vi "DAQAI_ws.vi"(2 "rate":dbl=1000.0, 3 "number of samples":i32=1000, 4 "timeout (s)":dbl=10.0 format="%0.2f", 5 "error in":errorcluster) -> (15 "data":dynamicdata(graph), 19 "error out":errorcluster)   [LabVIEW 2018]
doc: "Creates, edits, and runs tasks using NI-DAQmx. Refer to the NI-DAQmx Readme for a complete listing of devices NI-DAQmx supports.\n\nWhen you place this Express VI on the block diagram, the DAQ Assistant launches to create a new task. After you create a task, you can double-click the DAQ Assistant Express VI to edit that task. For continuous measurement or generation, place a while loop around the DAQ Assistant Express VI."
uses:
  AI channel settings.ctl
panel:
  in  "stop":bool
  in  "AI channel setting":T1={"device name"="Dev1", "physical channel"=["ai0", "ai1", "ai2", "ai3", "ai4", "ai5", "ai6", "ai7"], "channel name"=["Voltage_0", "Voltage_1", "Voltage_2", "Voltage_3", "Voltage_4", "Voltage_5", "Voltage_6", "Voltage_7"], "maximum value"=[10.0, 10.0, 10.0, 10.0, 10.0, 10.0, 10.0, 10.0], "minimum value"=[-10.0, -10.0, -10.0, -10.0, -10.0, -10.0, -10.0, -10.0], "units"=10348} {"units" items=["Volts"=10348, "From TEDS"=12516, "From Custom Scale"=10065]}
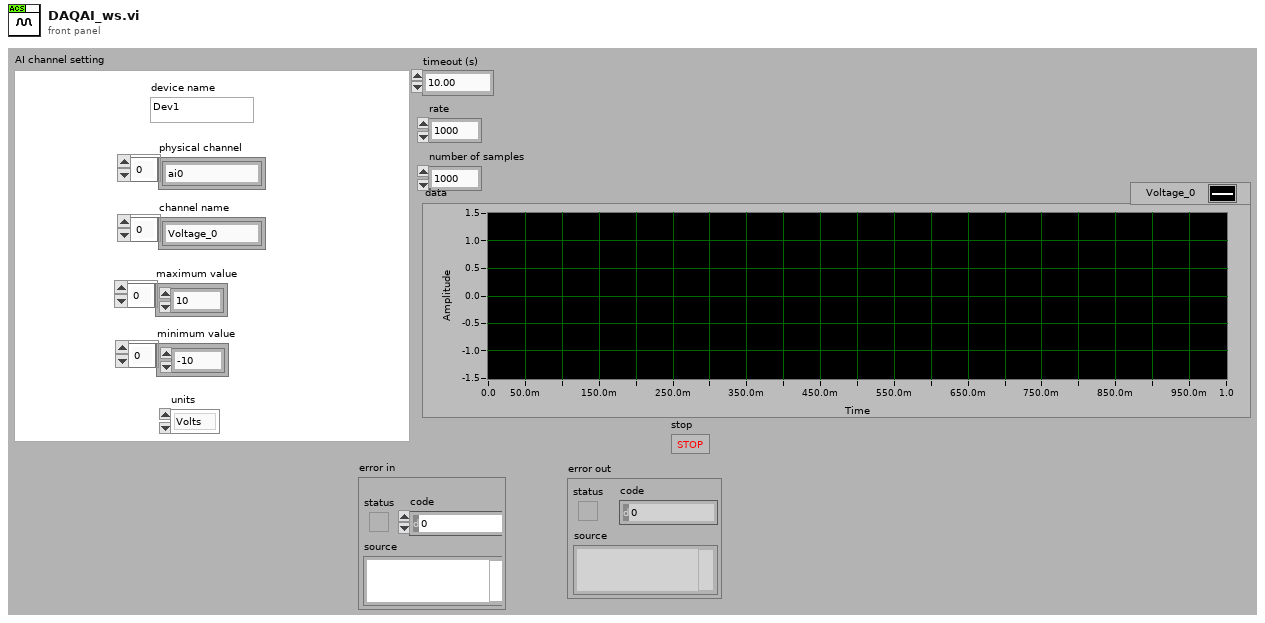
[diagram p1: front panel]
types:
  T1 = typedef "AI channel settings.ctl" = cluster{"device name":string, "physical channel":string[], "channel name":string[], "maximum value":dbl[], "minimum value":dbl[], "units":i32}
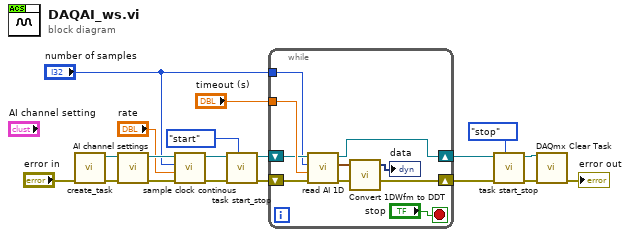
[diagram p0: block diagram]
diagram:
  n1 = call "create_task.vi"("error in (no error)"="error in") -> ("error out"=w16:errorcluster, "Refnum out"=w17:refnum<k21>)  [unwired: 9 in]
  n2 = call "AI channel settings.vi"("error in (no error)"=w16, "Refnum in"=w17) -> ("error out"=w14:errorcluster, "Refnum out"=w15:refnum<k21>)  [unwired: 8 in]
  n3 = call "sample clock continous.vi"("error in (no error)"=w14, "rate"="rate", "number of samples"="number of samples", "Refnum in"=w15) -> ("error out"=w9:errorcluster, "Refnum out"=w10:refnum<k21>)  [unwired: 6 in]
  n4 = call "task start_stop.vi"("Start/Stop"=enum16{"start", "stop"}."start", "Error In"=w9, "task/channels in"=w10) -> ("Error Out"=w7:errorcluster, "task out"=w8:refnum<k21>)  [unwired: 7 in]
  n5 = while {
    tunnel: "timeout (s)" -> [w27]
    tunnel: "number of samples" -> [w21]
    shift-right: [w23] -> w6
    shift-left: w8 -> [w25]
    shift-right: [w22] -> w4
    shift-left: w7 -> [w24]
    stop <- "stop" stop-if-true
    n6 = call "read AI 1D.vi"("error in (no error)"=w24, "timeout (s)"=w27, "number of samples per channel"=w21, "Refnum in"=w25) -> ("error out"=w22:errorcluster, "data"=w28:waveform(dbl)[], "Refnum out"=w23:refnum<k21>)  [unwired: 5 in]
    n7 = call <vilib>:"Convert 1DWfm to DDT.vi"("Array of Waveforms"=w28) -> ("Dynamic Data Type"=→"data":dynamicdata)  [unwired: 3 in]
  }
  n8 = call "task start_stop.vi"("Start/Stop"=enum16{"start", "stop"}."stop", "Error In"=w4, "task/channels in"=w6) -> ("Error Out"=w3:errorcluster, "task out"=w2:refnum<k21>)  [unwired: 7 in]
  n9 = call <vilib>:"DAQmx Clear Task.vi"("task in"=w2, "error in"=w3) -> ("error out"=→"error out":errorcluster)  [unwired: 13 in]
